vi "Base64url_Decode.vi"(10 "error in (no error)":errorcluster, 11 "Base64 URL String":string) -> (2 "error out":errorcluster, 3 "Decoded String":string)   [LabVIEW 2013, in "Serializer.Base64.lvclass"]
doc: "Decodes a <B>Base64 URL</B> encoded string."
uses:
  Serializer.Base64.lvclass
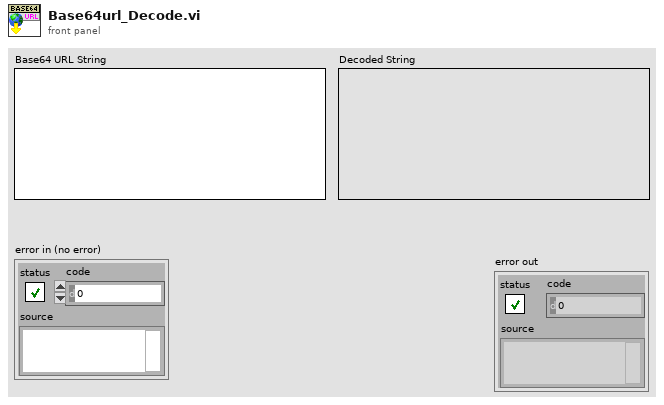
[diagram p1: front panel]
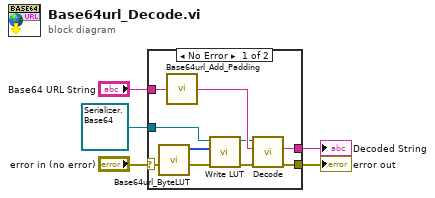
[diagram p0: block diagram]
diagram:
  n1 = case shown="No Error" "error in (no error)" {
    selector: "error in (no error)" -> [w8 w15]
    tunnel: "Base64 URL String" -> [w12 _]
    tunnel: [w14 w15] -> w3
    tunnel: refnum<class "Serializer.Base64.lvclass"> refnum ("Serializer.Base64.lvclass") -> [w10 _]
    tunnel: [w13 _] -> w1
    frame No Error {
      n2 = call "Base64url_ByteLUT.vi"() -> ("Base64 URL LUT"=w9:u32[])  [unwired: 11 in]
      n3 = call "Base64url_Add_Padding.vi"("Base64url string"=w12) -> ("Base64 string"=w11:string)
      n4 = call "Write LUT.vi"("error in (no error)"=w8, "LUT"=w9, "Serializer.Base64 in"=w10) -> ("error out"=w7:errorcluster, "Serializer.Base64 out"=w6:refnum<class "Serializer.Base64.lvclass">)  [unwired: 7 in]
      n5 = call "Decode.vi"("error in (no error)"=w7, "Base64 String"=w11, "Serializer.Base64 in"=w6) -> ("error out"=w14:errorcluster, "decoded string"=w13:string)  [unwired: 6 in, 1 out]
    }
    frame Error {
    }
  }
  "Decoded String" <- w1
  "error out" <- w3
